vi "LaunchClient.vi"() -> ()   [LabVIEW 2023]
uses:
  TCP_Client_Window/TCP_Client_Window.lvclass
  TCP_Client_Window Messages/UpdateWindowTitle Msg/UpdateWindowTitle Msg.lvclass/UpdateWindowTitle Msg.ctl
  <vilib>/ActorFramework/Message Enqueuer/Message Enqueuer.lvclass/Message Enqueuer.ctl
  <vilib>/ActorFramework/Message Enqueuer/Enqueue.vi
  TCP_Client_Window Messages/UpdateWindowTitle Msg/UpdateWindowTitle Msg.lvclass
  <vilib>/ActorFramework/Stop Msg/Stop Msg.lvclass
  <vilib>/ActorFramework/Message Priority Queue/Priority Enqueue.vi
  <vilib>/ActorFramework/Actor/Actor.lvclass
panel:
  out "error out":errorcluster
  in  "Stop Button":bool
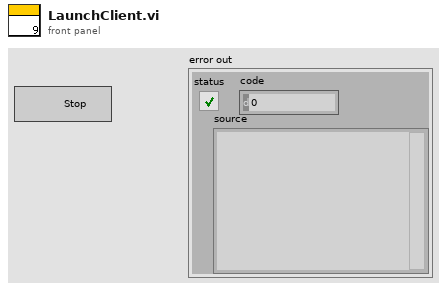
[diagram p1: front panel]
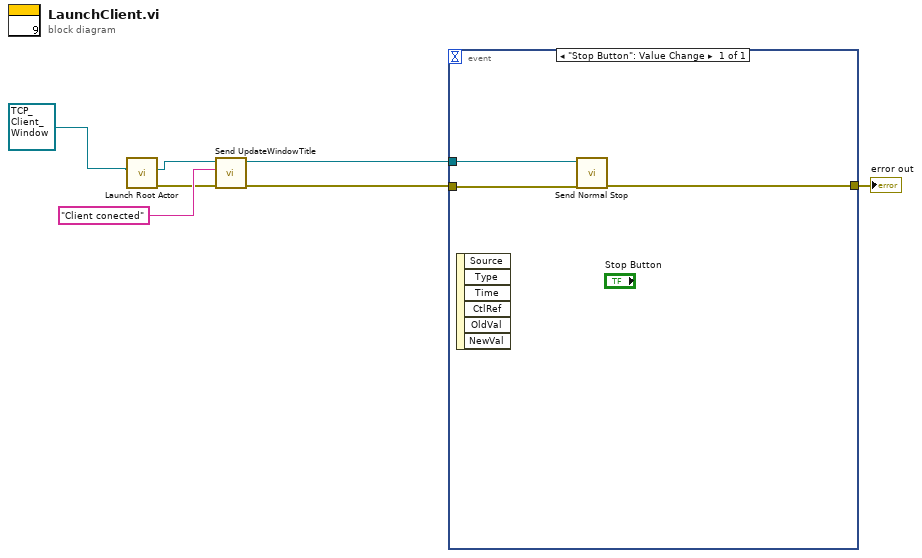
[diagram p0: block diagram]
diagram:
  n1 = call <vilib>:"Launch Root Actor.vi"("Actor"=refnum<class "TCP_Client_Window.lvclass"> refnum ("TCP_Client_Window.lvlib:TCP_Client_Window.lvclass")) -> ("error out"=w3:errorcluster, "Actor's Enqueuer"=w4:refnum<class "Message Enqueuer.lvclass">)  [unwired: 9 in]
  n2 = call "Send UpdateWindowTitle.vi"("error in (no error)"=w3, "WindowTitle"="Client conected", "Message Enqueuer"=w4) -> ("error out"=w1:errorcluster, "Message Enqueuer out"=w2:refnum<class "Message Enqueuer.lvclass">)  [unwired: 7 in]
  n3 = event shown="[0] \"Stop Button\": Value Change" {
    selector: _ -> [_]
    dyn-events: _ -> [_]
    timeout: _ -> [_]
    tunnel: w2 -> [w10]
    tunnel: w1 -> [w9]
    tunnel: [w8] -> w7
    event "Stop Button": Value Change {
      n4 = event-data() -> ()  [unwired: 1 in, 6 out]
      n5 = call <vilib>:"Send Normal Stop.vi"("error in (no error)"=w9, "Message Enqueuer"=w10) -> ("error out"=w8:errorcluster)  [unwired: 9 in]
    }
  }
  "error out" <- w7
